vi "Find Onset by SD.vi"(5 "Quiet Rewind (0.03s)":dbl=0.03, 7 "Quiet Threshold (500)":dbl=500.0, 9 "#SDs (3)":dbl=3.0, 10 "Sample Rate (Hz)":dbl, 11 "Data":dbl[](array[numeric])) -> (2 "Onset (idx)":i32, 3 "Onset (s)":dbl)   [LabVIEW 2016]
uses:
  <vilib>/Analysis/NI_AALBase.lvlib
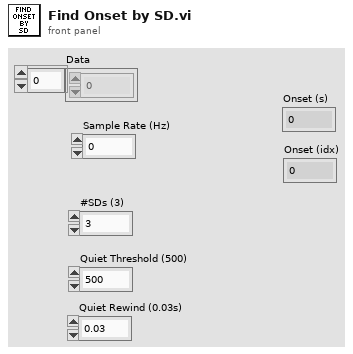
[diagram p1: front panel]
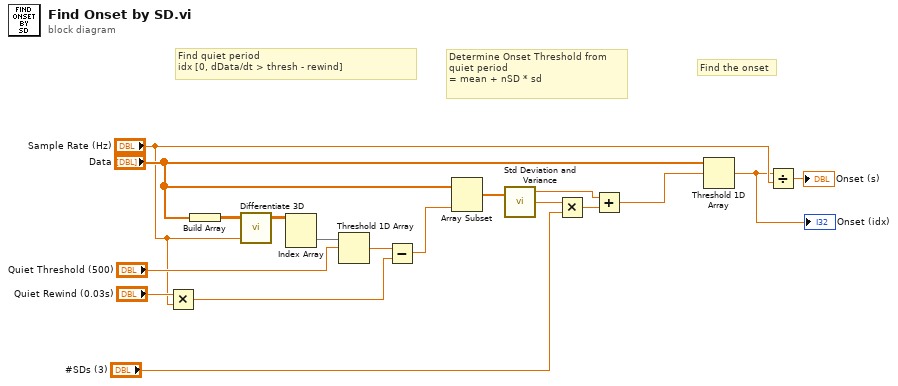
[diagram p0: block diagram]
diagram:
  # "Find the onset"
  # "Determine Onset Threshold from quiet period\n= mean + nSD * sd"
  # "Find quiet period\nidx [0, dData/dt > thresh - rewind]"
  n1 = Multiply(x="Quiet Rewind (0.03s)", y="Sample Rate (Hz)") -> (x*y=w12:dbl)
  n2 = Build Array("Data") -> (w18:dbl[][])
  n3 = call "Differentiate 3D.vi"("Sample Rate 4"="Sample Rate (Hz)", "Data (in)"=w18) -> ("Data (differentiated)"=w17:dbl[][])  [unwired: 3 in]
  n4 = Index Array(array=w17) -> (element=w16:dbl[])  [unwired: 2 in]
  n5 = Threshold 1D Array(2:"Quiet Threshold (500)", 3:w16) -> (0:w13:dbl)  [unwired: 1 in]
  n6 = Subtract(x=w13, y=w12) -> (x-y=w11:dbl)
  n7 = Array Subset(array="Data", length=w11) -> (w10:dbl[])  [unwired: 1 in]
  n8 = call <vilib>:"Std Deviation and Variance.vi"("X"=w10) -> ("mean"=w6:dbl, "standard deviation"=w9:dbl)  [unwired: 1 in, 1 out]
  n9 = Multiply(x=w9, y="#SDs (3)") -> (x*y=w7:dbl)
  n10 = Add(x=w6, y=w7) -> (x+y=w5:dbl)
  n11 = Threshold 1D Array(2:w5, 3:"Data") -> (0:w1:dbl)  [unwired: 1 in]
  "Onset (idx)" <- w1
  n12 = Divide(x=w1, y="Sample Rate (Hz)") -> (x/y=→"Onset (s)":dbl)
